vi "measuretime.vi"() -> ()   [LabVIEW 2021]
panel:
  out "total time":u32
  out "F(n)":u32
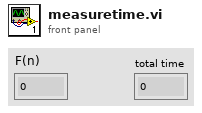
[diagram p1: front panel]
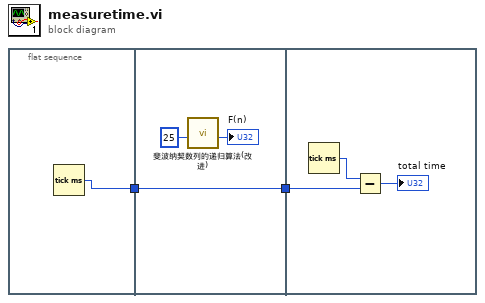
[diagram p0: block diagram]
diagram:
  n1 = flat-sequence {
    tunnel: [w3] -> w2
    tunnel: w2 -> [w4]
    tunnel: [w4] -> w1
    tunnel: w1 -> [w8]
    frame #0 {
      n2 = Tick Count (ms)() -> (millisecond timer value=w3:u32)
    }
    frame #1 {
      n3 = call "斐波纳契数列的递归算法(改进).vi"("n"=u32 25) -> ("F(n)"=→"F(n)":u32)  [unwired: 10 in]
    }
    frame #2 {
      n4 = Tick Count (ms)() -> (millisecond timer value=w9:u32)
      n5 = Subtract(x=w9, y=w8) -> (x-y=→"total time":u32)
    }
  }
